vi "補正系統.vi"(0 "Image In":T2, 1 "element":T1, 2 "Coordinate System In":T3 {"Measurement System"."Axis Reference" items=["Direct", "Indirect"]; "Measurement System"."Angle (deg)" format="%.2f"; "Measurement System"."Origin"."Y" format="%.2f"; "Measurement System"."Origin"."X" format="%.2f"; "Reference System"."Axis Reference" items=["Direct", "Indirect"]; "Reference System"."Angle (deg)" format="%.2f"; "Reference System"."Origin"."Y" format="%.2f"; "Reference System"."Origin"."X" format="%.2f"}, 3 "error Input":errorcluster, 4 "Mode":u16(ring) items=["Find Reference", "Update CoordSys"]) -> (7 "ImageOut":T2, 9 "Coordinate System Out":T3 {"Measurement System"."Axis Reference" items=["Direct", "Indirect"]; "Measurement System"."Angle (deg)" format="%.2f"; "Measurement System"."Origin"."Y" format="%.2f"; "Measurement System"."Origin"."X" format="%.2f"; "Reference System"."Axis Reference" items=["Direct", "Indirect"]; "Reference System"."Angle (deg)" format="%.2f"; "Reference System"."Origin"."Y" format="%.2f"; "Reference System"."Origin"."X" format="%.2f"}, 10 "error out":errorcluster)   [LabVIEW 2015]
uses:
  <vilib>/vision/Image Controls.llb/IMAQ Image.ctl
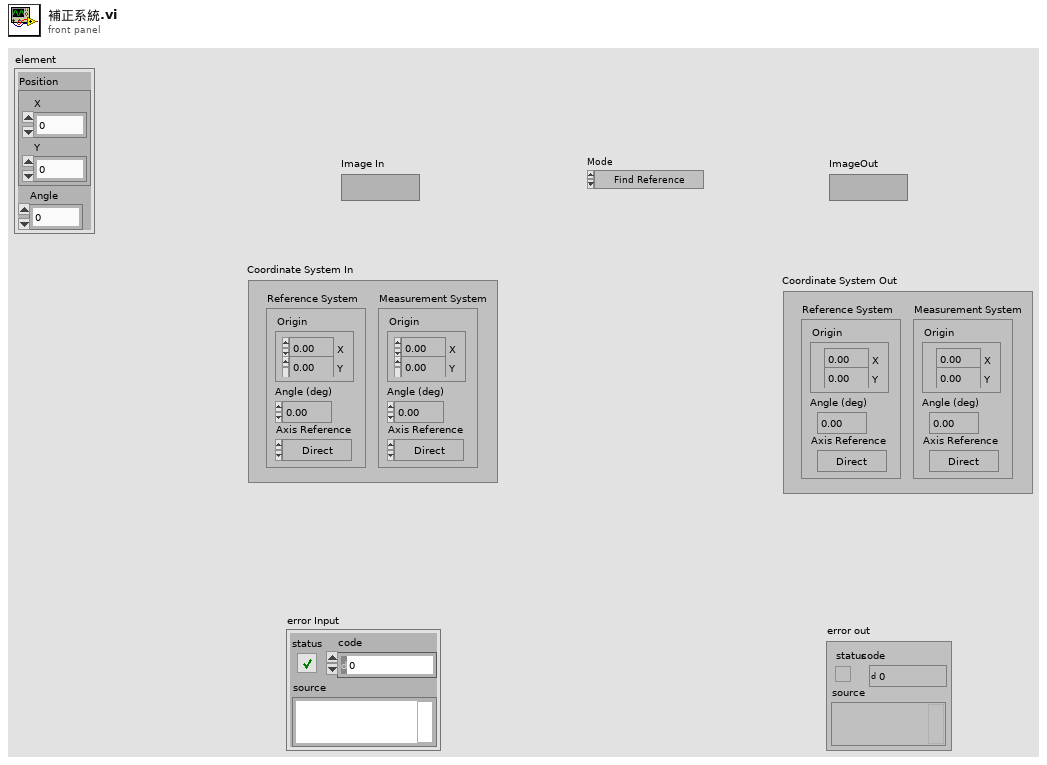
[diagram p1: front panel]
types:
  T1 = cluster{"Position":cluster{"X":sgl, "Y":sgl}, "Angle":dbl}
  T2 = typedef "IMAQ Image.ctl" = refnum<image>
  T3 = typedef "IMAQ Coordinate System" = cluster{"Reference System":cluster{"Origin":cluster{"X":sgl, "Y":sgl}, "Angle (deg)":sgl, "Axis Reference":u32}, "Measurement System":cluster{"Origin":cluster{"X":sgl, "Y":sgl}, "Angle (deg)":sgl, "Axis Reference":u32}}
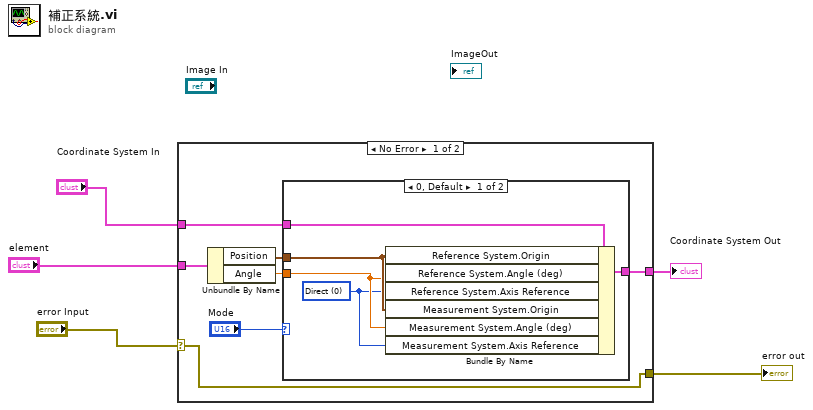
[diagram p0: block diagram]
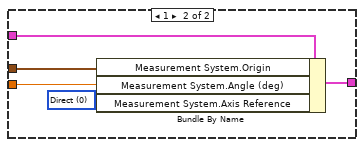
[diagram p2: hidden frame]
diagram:
  n1 = case shown="No Error" "error Input" {
    selector: "error Input" -> [w6 w23]
    tunnel: "element" -> [w12 _]
    tunnel: "Coordinate System In" -> [w11 w24]
    tunnel: [w7 w24] -> w5
    tunnel: [w6 w23] -> w2
    frame No Error {
      n2 = Unbundle By Name(w12) -> ("Position"=w10:cluster{"X":sgl, "Y":sgl}, "Angle"=w9:dbl)
      n3 = case shown="0, Default" "Mode" {
        tunnel: w10 -> [w15 w20]
        tunnel: [w17 w22] -> w7
        tunnel: w9 -> [w14 w19]
        tunnel: w11 -> [w16 w21]
        frame 0, Default {
          w13 = u32 0 items=["Direct", "Indirect"] ("Axis Reference")
          n4 = Bundle By Name(cluster=w16, "Reference System.Origin"=w15, "Reference System.Angle (deg)"=w14, "Reference System.Axis Reference"=w13, "Measurement System.Origin"=w15, "Measurement System.Angle (deg)"=w14, "Measurement System.Axis Reference"=w13) -> (w17:T3)
        }
        frame 1 {
          w18 = u32 0 items=["Direct", "Indirect"] ("Axis Reference")
          n5 = Bundle By Name(cluster=w21, "Measurement System.Origin"=w20, "Measurement System.Angle (deg)"=w19, "Measurement System.Axis Reference"=w18) -> (w22:T3)
        }
      }
    }
    frame Error {
    }
  }
  "Coordinate System Out" <- w5
  "error out" <- w2
